vi "get_size.vi"(8 "error in (no error)":errorcluster, 11 "Image in":refnum<class "Image.lvclass">) -> (0 "error out":errorcluster, 1 "y resolution":i32, 2 "x resolution":i32, 3 "Image out":refnum<class "Image.lvclass">, 4 "memory size (kB)":i32, 5 "physical size y":dbl, 6 "max resolution":i32, 7 "physical size x":dbl)   [LabVIEW 2010, in "Image.lvclass"]
uses:
  Image.lvclass
  storage_mode.ctl
  ErrorController/ErrorController/class_data.vi
  ErrorController/ErrorController/ErrorController.lvclass
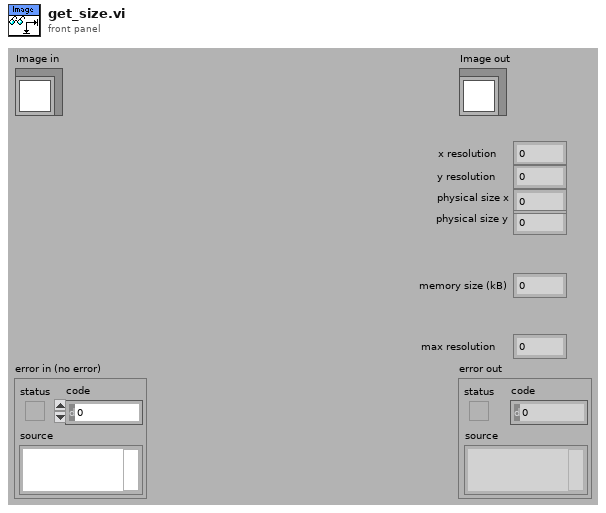
[diagram p1: front panel]
types:
  T1 = typedef "Image.lvclass/storage_mode.ctl" = enum16{"RAM", "disk"}
  T2 = typedef "IMAQ Image.ctl" = refnum<image>
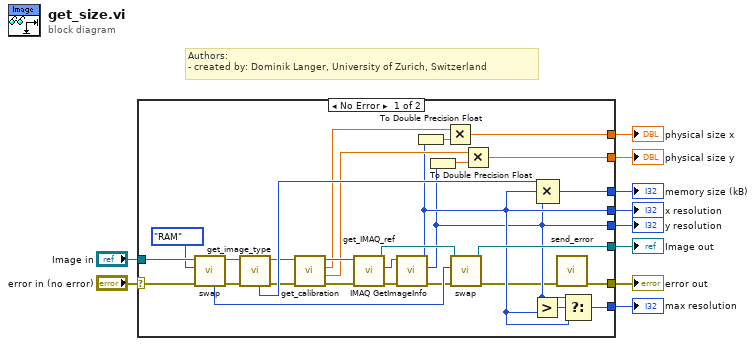
[diagram p0: block diagram]
diagram:
  # "Authors: \n- created by: Dominik Langer, University of Zurich, Switzerland"
  n1 = case shown="No Error" "error in (no error)" {
    selector: "error in (no error)" -> [w38 w41]
    tunnel: [w11 w41] -> w9
    tunnel: [w32 w40] -> w7
    tunnel: "Image in" -> [w39 w40]
    tunnel: [w16 _] -> w6
    tunnel: [w15 _] -> w5
    tunnel: [w31 _] -> w4
    tunnel: [w28 _] -> w3
    tunnel: [w14 _] -> w2
    tunnel: [w13 _] -> w1
    frame No Error {
      n2 = call-dynamic "swap.vi"("error in (no error)"=w38, "storage type target"=storage_mode."RAM", "Image in"=w39) -> ("error out"=w27:errorcluster, "Image out"=w26:refnum<class "Image.lvclass">, "previous storage mode"=w37:T1)  [unwired: 6 out]
      n3 = call-dynamic "get_image_type.vi"("error in (no error)"=w27, "Image.lvclass in"=w26) -> ("error out"=w24:errorcluster, "Image.lvclass out"=w23:refnum<class "Image.lvclass">, "bytes per pixel"=w25:i32)  [unwired: 6 in, 1 out]
      n4 = call "get_calibration.vi"("error in (no error)"=w24, "Image.lvclass in"=w23) -> ("error out"=w22:errorcluster, "y"=w19:dbl, "x"=w20:dbl, "Image.lvclass out"=w21:refnum<class "Image.lvclass">)  [unwired: 4 in, 2 out]
      n5 = call-dynamic "get_IMAQ_ref.vi"("error in (no error)"=w22, "Image.lvclass in"=w21) -> ("error out"=w34:errorcluster, "Image"=w30:T2, "Image.lvclass out"=w35:refnum<class "Image.lvclass">)  [unwired: 7 out]
      n6 = call "IMAQ GetImageInfo"("error in (no error)"=w34, "Image"=w30) -> ("error out"=w33:errorcluster, "Y Resolution"=w15:i32, "X Resolution"=w16:i32)  [unwired: 2 in, 5 out]
      n7 = To Double Precision Float(number=w16) -> (double precision float=w17:dbl)
      n8 = To Double Precision Float(number=w15) -> (double precision float=w18:dbl)
      n9 = Multiply(x=w20, y=w17) -> (x*y=w14:dbl)
      n10 = call-dynamic "swap.vi"("error in (no error)"=w33, "storage type target"=w37, "Image in"=w35) -> ("error out"=w12:errorcluster, "Image out"=w32:refnum<class "Image.lvclass">)  [unwired: 7 out]
      n11 = Multiply(x=w19, y=w18) -> (x*y=w13:dbl)
      n12 = Greater?(x=w15, y=w16) -> (0:w29:bool)
      n13 = Compound Arithmetic op=MULTIPLY(w25, w16, w15) -> (w31:i32)
      n14 = call "send_error.vi"("error in (no error)"=w12) -> ("error out"=w11:errorcluster)  [unwired: 10 in]
      n15 = Select(t=w15, s=w29, f=w16) -> (s? t:f=w28:i32)
    }
    frame Error {
    }
  }
  "error out" <- w9
  "Image out" <- w7
  "x resolution" <- w6
  "y resolution" <- w5
  "memory size (kB)" <- w4
  "max resolution" <- w3
  "physical size x" <- w2
  "physical size y" <- w1
